vi "Main Loop.vi"(8 "error in (no error)":errorcluster, 10 "Chart Notifier":refnum<notifier>, 11 "Message Queues":T1) -> (0 "error out":errorcluster)   [LabVIEW 2018, in "Scale Module.lvlib" / "Scale Module Engine.lvlib"]
uses:
  Scale Module Engine.lvlib
  Scale Message Queues.ctl
  support/Message Queue/Message Cluster.ctl
  State Cluster.ctl
  State Enum.ctl
  Feed Module/Controls/Scale Module Settings Cluster.ctl
  Mettler Toledo/Controls/Settings Cluster.ctl
  Feed Module/Controls/Scale Module Display.ctl
  <vilib>/Platform/TimedLoop/XDataNode/timing_clust.ctl
  <vilib>/Platform/TimedLoop/XDataNode/nitl_modes.ctl
  <vilib>/Platform/TimedLoop/XDataNode/wakeup.ctl
  Tag VIs/Tag FGV Operation Enum.ctl
  support/Message Queue/Enqueue Message (Single).vi
  <vilib>/Utility/error.llb/Error Cluster From Error Code.vi
  <vilib>/Platform/TimedLoop/XDataNode/XDataNode.xnode
  <vilib>/ErrorRing/Error Ring.xnode
  support/Message Queue/Message Queue.lvlib
  <vilib>/Platform/TimedLoop/XDataNode/XDNodeRunTimeDep.lvlib
  Scale Module.lvlib
  Mettler Toledo/Mettler Toledo.lvlib
  Shared Variables/Dynamic Shared Variables.lvlib
  support/Support Library.lvlib
panel:
  out "Period (s)":dbl format="%_4g"
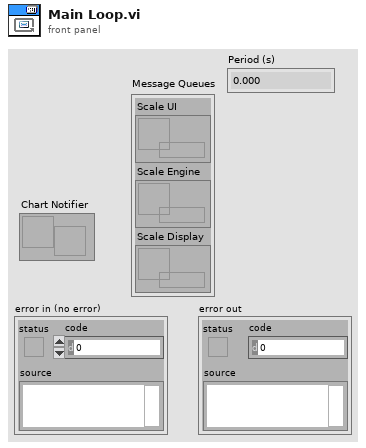
[diagram p1: front panel]
types:
  T1 = typedef "Scale Module.lvlib/Scale Message Queues.ctl" = cluster{"Scale UI":refnum<queue>, "Scale Engine":refnum<queue>, "Scale Display":refnum<queue>}
  T2 = typedef "Scale Module.lvlib/Scale Module Engine.lvlib/State Cluster.ctl" = cluster{"State":T3, "Start Time":timestamp, "Configuration":T4, "Current Time":timestamp, "First Iteration":bool, "Data":cluster{"Scale Read(g)":dbl}, "Process Name":string, "Log Started":bool}
  T3 = typedef "Scale Module.lvlib/Scale Module Engine.lvlib/State Enum.ctl" = enum16{"Measuring", "Idle"}
  T4 = typedef "Scale Module.lvlib/Scale Module Settings Cluster.ctl" = cluster{"Cycle Period":dbl, "Mettler":T5, "Scale Type":string}
  T5 = typedef "Mettler Toledo.lvlib/Settings Cluster.ctl" = cluster{"VISA resource name":refnum<visa-resource-name>, "Simulated?":bool}
  T6 = typedef "XDNodeRunTimeDep.lvlib/timing_clust.ctl" = cluster{"Expected End [f-1]":u64, "Actual End [f-1]":u64, "Finished Late? [f-1]":bool, "Expected End [i-1]":u64, "Actual End [i-1]":u64, "Finished Late? [i-1]":bool, "Expected Start [i]":u64, "Actual Start [i]":u64, "Expected Start [f]":u64, "Actual Start [f]":u64, "Source Name":string, "Structure Name":string, "Period":i64, "Deadline":i64, "Offset":i64, "Start":i64, "Priority":i32, "Timeout":i32, "Mode":T7, "Wakeup Reason":T8, "Error":errorcluster, "Source Type":string, "Secondary Source Type":string, "Global End Time":u64, "Global Start Time":u64, "Frame Duration":u64, "Iteration Duration":u64, "Assigned CPU":i32, "I/O Scan Engine Mode":u32}
  T7 = typedef "XDNodeRunTimeDep.lvlib/nitl_modes.ctl" = enum32{"No Change", "Process missed periods, maintain original phase", "Discard missed periods, maintain original phase", "Process missed periods, ignore original phase", "Discard missed periods, ignore original phase"}
  T8 = typedef "XDNodeRunTimeDep.lvlib/wakeup.ctl" = enum32{"Normal", "Aborted", "Asynchronous wakeup", "Timing source error", "Timed loop error", "Timeout"}
  T9 = cluster{"enable? (F)":bool, "name":string, "alarm on":bool, "priority":u32, "ack type":enum16{"Auto", "User", "None", "Each Occurrence"}, "area":string, "description":string, "log? (T)":bool}
  T10 = typedef "Tag FGV Operation Enum.ctl" = enum16{"Init", "Set Notification Queue", "Create Tag", "Commit", "Write Tag (Numeric)", "Write Tag (Boolean)", "Read All Tags", "Read One Tag", "Delete Tag Category", "Set Alarm Parameters (Numeric)", "Set Alarm Parameters (Boolean)", "Enable All Alarms", "Disable All Alarms", "Delete All Tags", "Read Alarms", "Ack Alarm", "Read Alarm Parameters (Numeric)", "Read Alarm Parameters (Boolean)"}
  T11 = enum32{"u32BitField", "bool", "double", "string", "int8", "uint8", "int16", "uint16", "int32", "uint32", "int64", "uint64", "single", "double waveform", "int16 waveform", "array of boolean", "array of int8", "array of uint8", "array of int16", "array of uint16", "array of int32", "array of uint32", "array of int64", "array of uint64", "array of single", "array of double", "array of double waveform", "array of int16 waveform", "array of string", "variant", "timestamp", "fixed point", "custom"}
  T12 = typedef "Scale Module.lvlib/Scale Module Display.ctl" = cluster{"Scale Value":dbl, "Cycle Period":dbl}
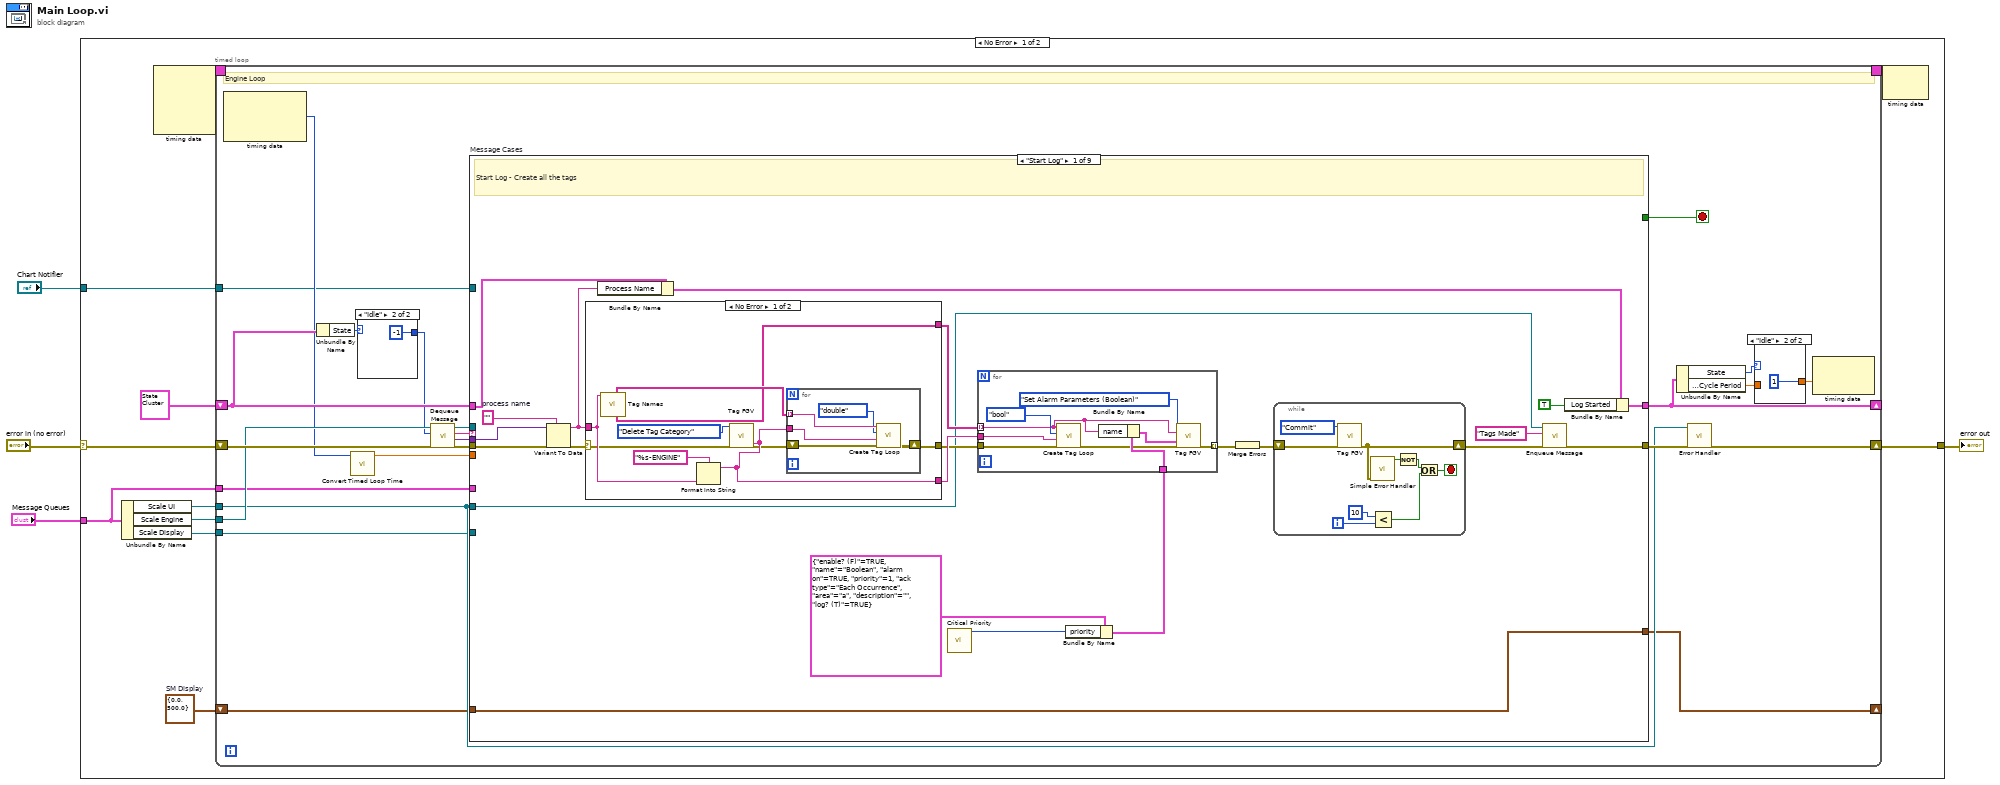
[diagram p0: block diagram]
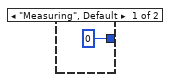
[diagram p3: hidden frame]
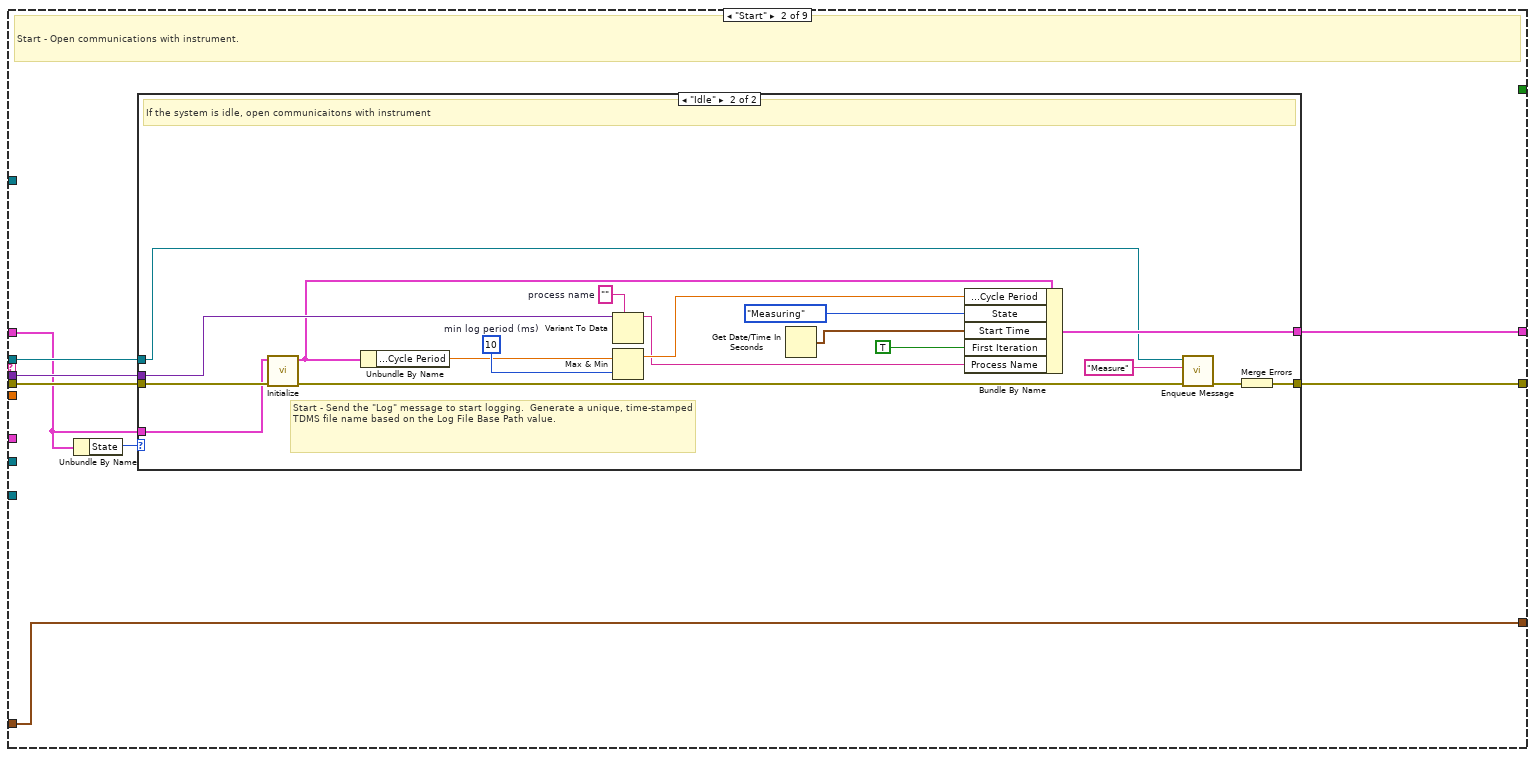
[diagram p5: hidden frame]
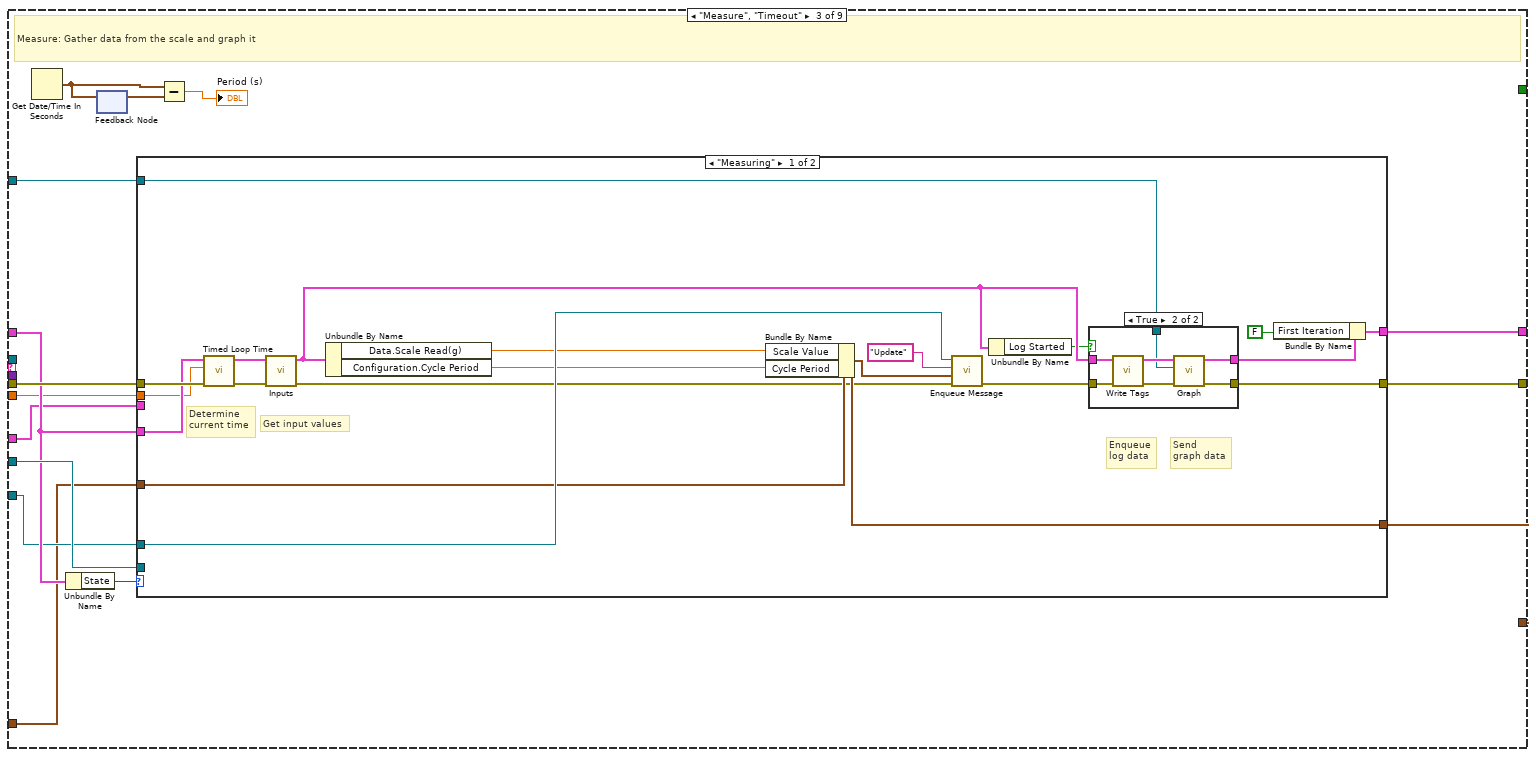
[diagram p7: hidden frame]
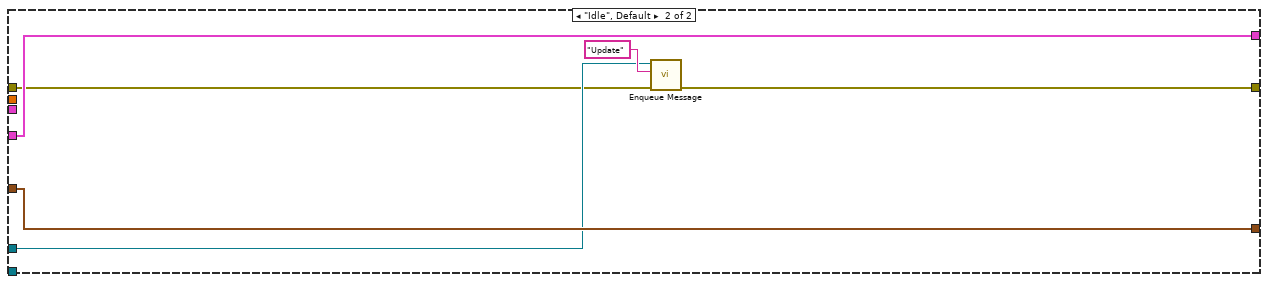
[diagram p9: hidden frame]
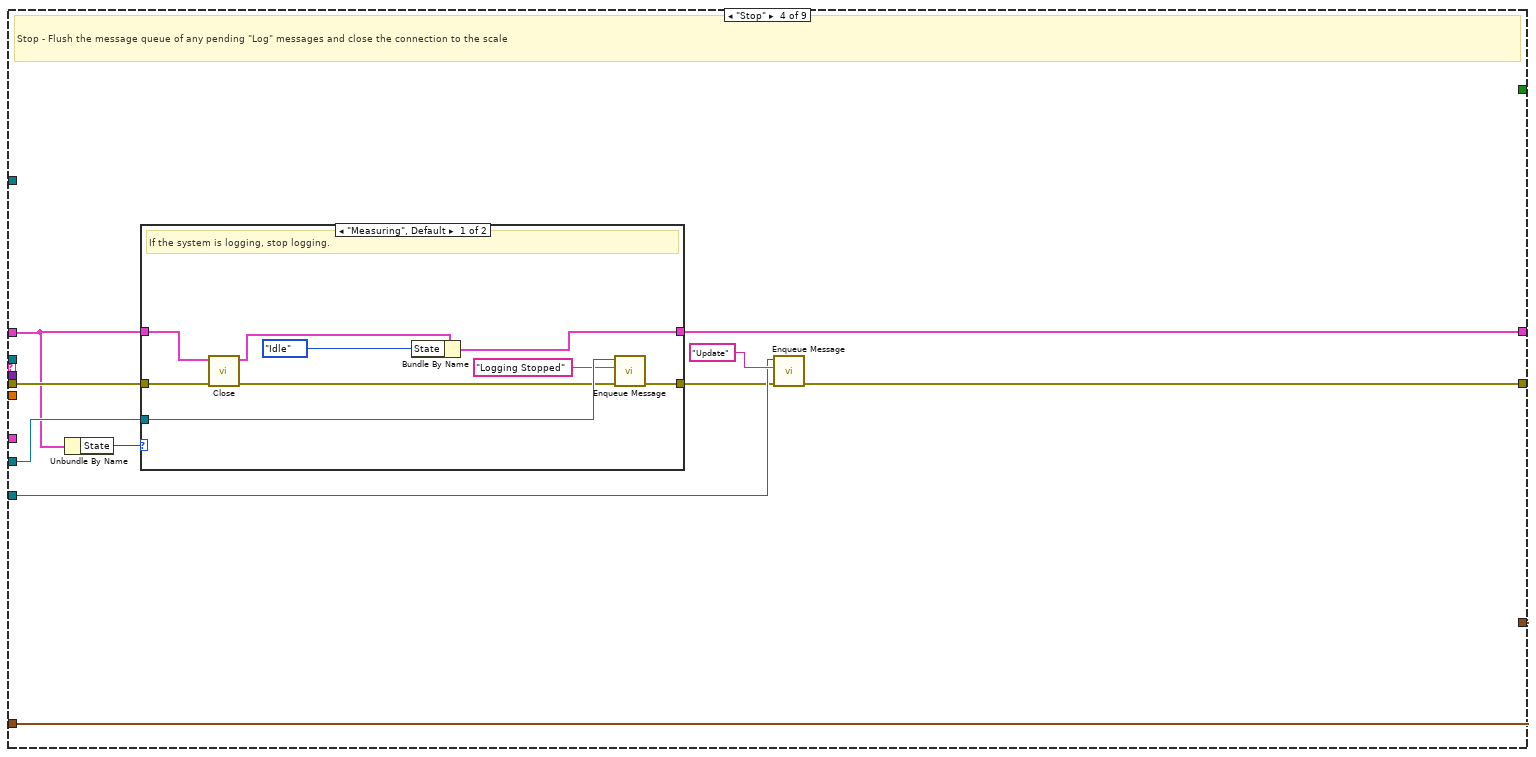
[diagram p10: hidden frame]
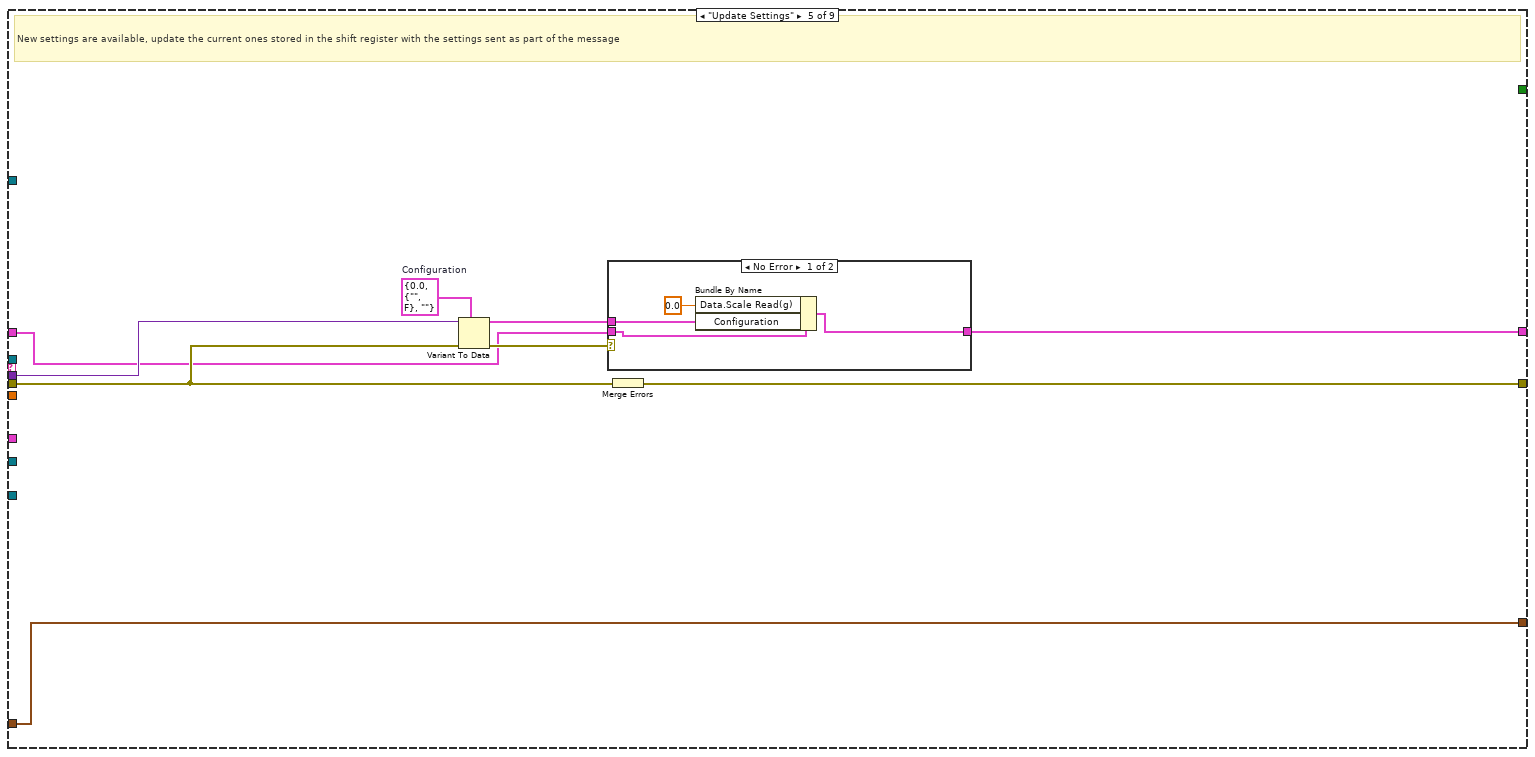
[diagram p12: hidden frame]
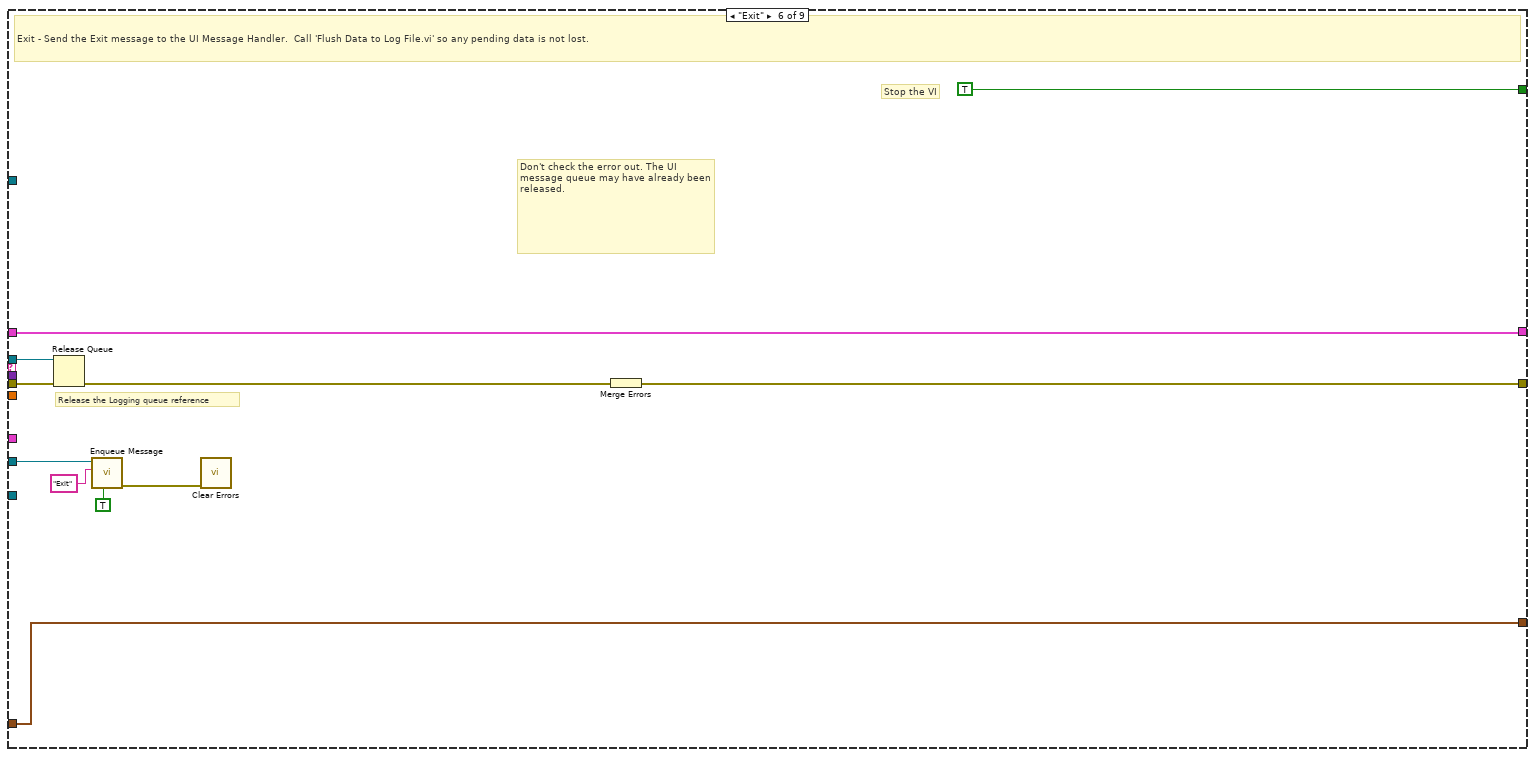
[diagram p14: hidden frame]
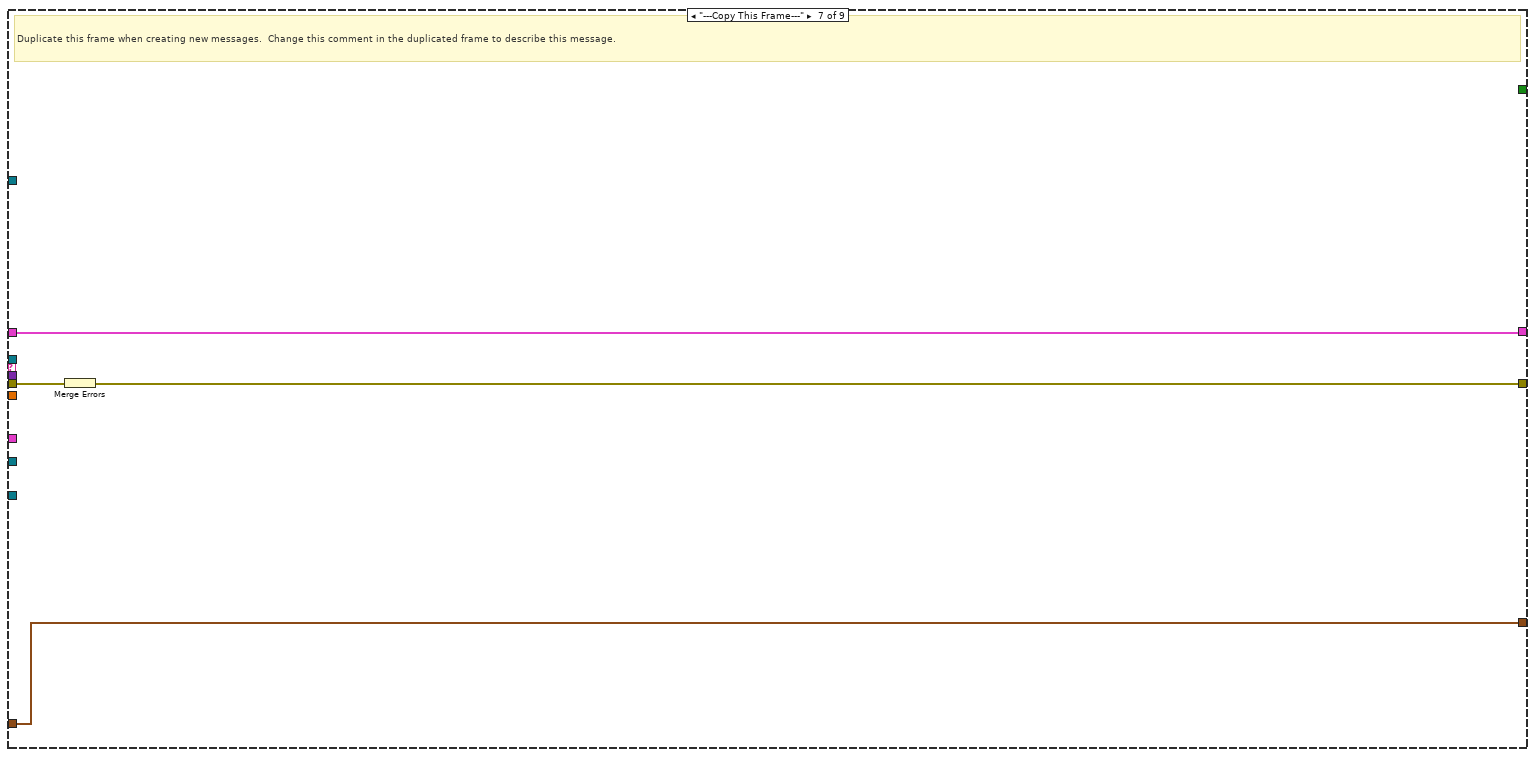
[diagram p15: hidden frame]
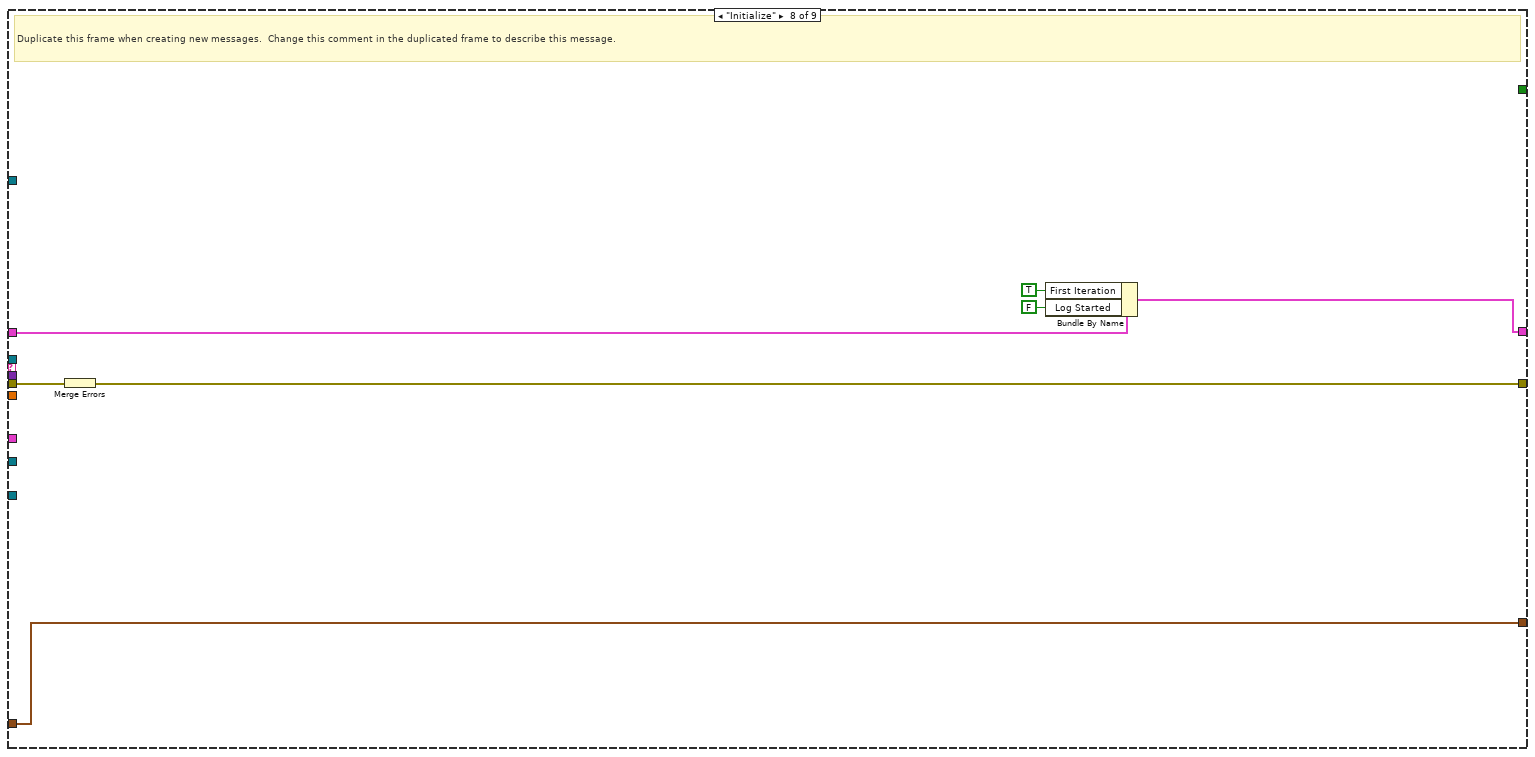
[diagram p16: hidden frame]
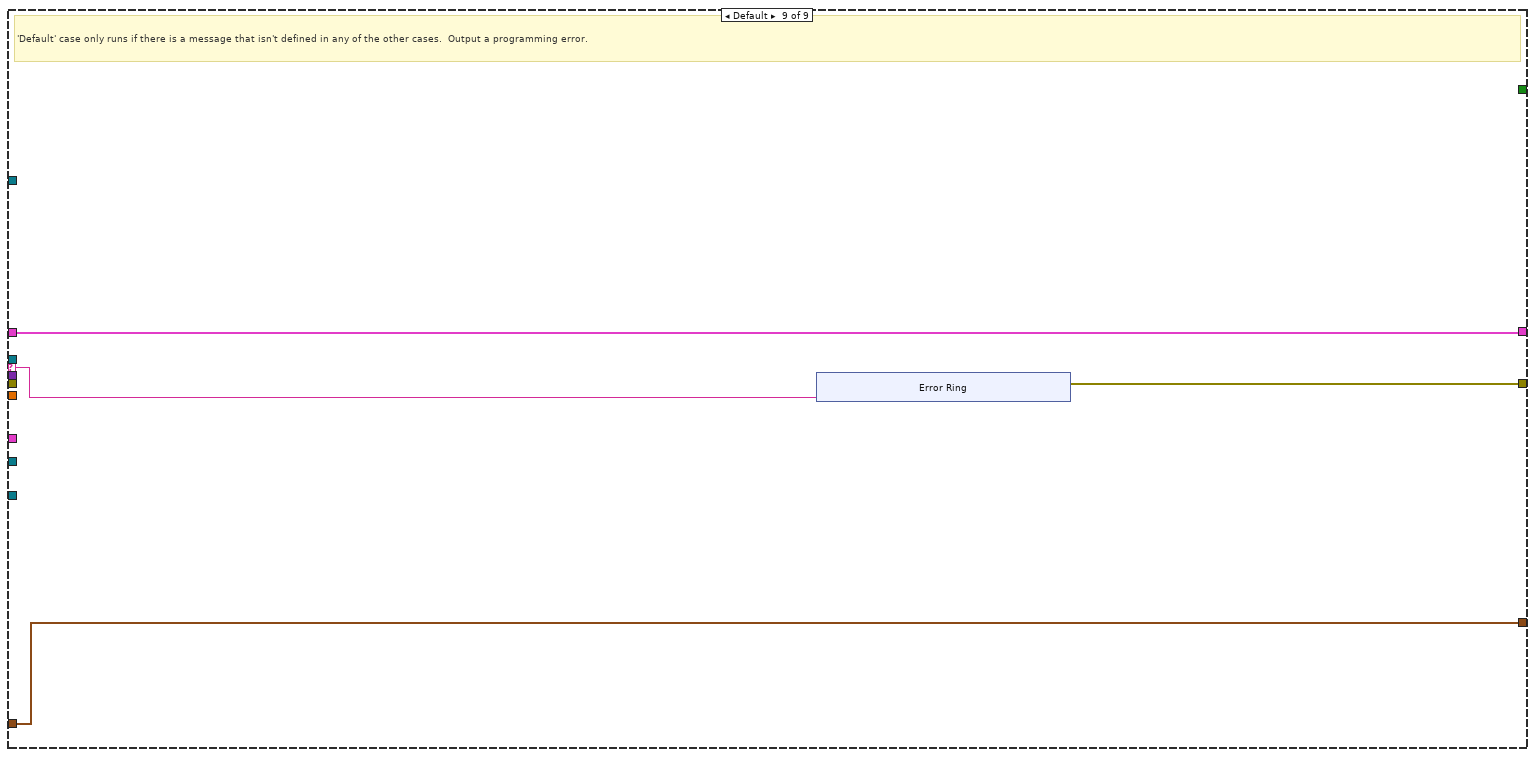
[diagram p17: hidden frame]
diagram:
  n1 = case shown="No Error" "error in (no error)" {
    selector: "error in (no error)" -> [w14 w252]
    tunnel: "Message Queues" -> [w9 _]
    tunnel: [w15 w252] -> w3
    tunnel: "Chart Notifier" -> [w7 _]
    frame No Error {
      w5 = T12 {"Scale Value"=0.0, "Cycle Period"=500.0}  # SM Display
      n2 = Unbundle By Name(w9) -> ("Scale UI"=w13:refnum<queue>, "Scale Engine"=w8:refnum<queue>, "Scale Display"=w6:refnum<queue>)
      n3 = node-c288() -> (w11:T6)  [unwired: 4 in]
      n4 = timed-loop {
        tunnel: w8 -> [w33]
        shift-right: [w17] -> _
        shift-left: T2 {"State"=enum."Idle", "Start Time"=timestamp(0 s since 1904-01-01), "Configuration"={"Cycle Period"=0.0, "Mettler"={"VISA resource name"="", "Simulated?"=FALSE}, "Scale Type"=""}, "Current Time"=timestamp(0 s since 1904-01-01), "First Iteration"=FALSE, "Data"={"Scale Read(g)"=0.0}, "Process Name"="", "Log Started"=FALSE} -> [w29]
        shift-right: [w31] -> w15
        shift-left: w14 -> [w38]
        tunnel: w13 -> [w30]
        timing: w11 -> [_]
        timing-out: [_] -> w10
        tunnel: w9 -> [w21]
        tunnel: w7 -> [w20]
        tunnel: w6 -> [w19]
        shift-right: [w18] -> _
        shift-left: w5 -> [w16]
        stop <- w39 stop-if-true
        # "Engine Loop"
        n5 = node-c288() -> (w23:i64)  [unwired: 1 in, 2 out]
        n6 = Unbundle By Name(w29) -> ("State"=w28:T3)
        n7 = call "Convert Timed Loop Time.vi"("Actual Start [i]"=w23) -> ("ET since start (s)"=w22:dbl)  [unwired: 10 in]
        n8 = case shown="\"Idle\"" w28 {
          tunnel: [0 ("timeout in ms (-1)") -1 ("timeout in ms (-1)")] -> w27
          frame "Measuring", Default {
          }
          frame "Idle" {
          }
        }
        n9 = call "Dequeue Message.vi"("error in (no error)"=w38, "timeout in ms (-1)"=w27, "Message Queue"=w33) -> ("error out"=w37:errorcluster, "Message Data"=w35:variant, "Message"=w36:string, "dup Message Queue"=w34:refnum<queue>)  [unwired: 5 in]
        n10 = case "Message Cases" shown="\"Start Log\"" w36 {
          selector: w36 -> [_ _ _ _ _ _ _ _ w241]
          tunnel: w34 -> [_ w110 _ _ _ w221 _ _ _]
          tunnel: w37 -> [w65 w109 w143 w191 w209 w224 w231 w238 _]
          tunnel: [w52 w111 w144 w182 w211 w226 w230 w237 w242] -> w32
          tunnel: w29 -> [w64 w106 w142 w188 w207 w217 w228 w235 w239]
          tunnel: [_ _ _ _ _ TRUE _ _ _] -> w39
          tunnel: w35 -> [w66 w107 _ _ w210 _ _ _ _]
          tunnel: w30 -> [w51 _ w145 w190 _ w225 _ _ _]
          tunnel: w22 -> [_ _ w141 _ _ _ _ _ _]
          tunnel: w21 -> [_ _ w140 _ _ _ _ _ _]
          tunnel: w20 -> [_ _ w136 _ _ _ _ _ _]
          tunnel: w19 -> [_ _ w135 w184 _ _ _ _ _]
          tunnel: w16 -> [w70 w105 w134 w187 w204 w218 w229 w236 w240]
          tunnel: [w70 w105 w133 w187 w204 w218 w229 w236 w240] -> w18
          tunnel: [w55 w104 w132 w186 w203 w217 w228 w232 w239] -> w17
          frame "Start Log" {
            w69 = ""  # process name
            # "Start Log - Create all the tags"
            n11 = Variant To Data(error in=w65, type=w69, Variant=w66) -> (data=w67:string, error out=w68:errorcluster)
            n12 = case shown="No Error" w68 {
              selector: w68 -> [w91 w103]
              tunnel: [w97 w103] -> w58
              tunnel: w67 -> [w95 _]
              tunnel: [w90 _] -> w60
              tunnel: [w93 _] -> w59
              frame No Error {
                n13 = call "Tag Names.vi"("Process Name"=w95) -> ("All Boolean Tags"=w93:string[], "All  Numeric Tags"=w94:string[])  [unwired: 8 in, 1 out]
                n14 = Format Into String(format string="%s-ENGINE", w95) -> (resulting string=w90:string)  [unwired: 2 in, 1 out]
                n15 = call "Tag FGV.vi"("Operation"=Tag_FGV_Operation_Enum."Delete Tag Category", "error in (no error)"=w91, "Tag Category"=w90) -> ("error out"=w89:errorcluster)  [unwired: 5 in, 7 out]
                n16 = for {
                  shift-right: [w102] -> w97
                  shift-left: w89 -> [w101]
                  tunnel: w90 -> [w98]
                  tunnel: w94 -> [w100] mode=indexing
                  n17 = call "Create Tag Loop.vi"("error in (no error)"=w101, "Tag Category"=w98, "data type"=T11."double", "Tag Name"=w100) -> ("error out"=w102:errorcluster)  [unwired: 7 in]
                }
              }
              frame Error {
              }
            }
            n18 = Bundle By Name(cluster=w64, "Process Name"=w67) -> (w56:T2)
            n19 = call "Critical Priority.vi"() -> ("critical priority"=w62:i32)  [unwired: 11 in]
            n20 = Bundle By Name(cluster=T9 {"enable? (F)"=TRUE, "name"="Boolean", "alarm on"=TRUE, "priority"=1, "ack type"=enum."Each Occurrence", "area"="a", "description"="", "log? (T)"=TRUE} ("Boolean alarm settings"), "priority"=w62) -> (w61:T9)
            n21 = for {
              tunnel: w61 -> [w88]
              tunnel: [w80] -> w57 mode=indexing
              tunnel: w59 -> [w82] mode=indexing
              tunnel: w60 -> [w85]
              tunnel: w58 -> [w87]
              n22 = call "Create Tag Loop.vi"("error in (no error)"=w87, "Tag Category"=w85, "data type"=T11."bool", "Tag Name"=w82) -> ("error out"=w81:errorcluster)  [unwired: 7 in]
              n23 = Bundle By Name(cluster=w88, "name"=w82) -> (w83:T9)
              n24 = call "Tag FGV.vi"("Operation"=Tag_FGV_Operation_Enum."Set Alarm Parameters (Boolean)", "Tag Name"=w82, "Data"=w83, "error in (no error)"=w81) -> ("error out"=w80:errorcluster)  [unwired: 4 in, 7 out]
            }
            n25 = Merge Errors(w57) -> (w49:errorcluster)
            n26 = while {
              shift-right: [w71] -> w50
              shift-left: w49 -> [w72]
              i -> [w78]
              stop <- w74 stop-if-true
              n27 = call "Tag FGV.vi"("Operation"=Tag_FGV_Operation_Enum."Commit", "error in (no error)"=w72) -> ("error out"=w71:errorcluster)  [unwired: 6 in, 7 out]
              n28 = call <vilib>:"Simple Error Handler.vi"("error in (no error)"=w71) -> ("error?"=w79:bool)  [unwired: 4 in, 4 out]
              n29 = Less?(x=10, y=w78) -> (x < y?=w75:bool)
              n30 = Not(x=w79) -> (.not. x?=w76:bool)
              n31 = Or(x=w76, y=w75) -> (x .or. y?=w74:bool)
            }
            n32 = call-poly "Enqueue Message.vi"("error in (no error)"=w50, "Message"="Tags Made", "Message Queue"=w51) -> ("error out"=w52:errorcluster)  [unwired: 7 in, 1 out]
            n33 = Bundle By Name(cluster=w56, "Log Started"=TRUE) -> (w55:T2)
          }
          frame "Start" {
            # "Start - Open communications with instrument."
            n34 = Unbundle By Name(w106) -> ("State"=w108:T3)
            n35 = case shown="\"Idle\"" w108 {
              tunnel: [w112 w131] -> w111
              tunnel: w110 -> [_ w122]
              tunnel: w109 -> [w112 w119]
              tunnel: w106 -> [w113 w118]
              tunnel: [w113 w129] -> w104
              tunnel: w107 -> [_ w116]
              frame "Measuring", Default {
                # "The system is already running. Ignore the \"Start\" message."
              }
              frame "Idle" {
                w117 = ""  # process name
                w126 = 10  # min log period (ms)
                # "Start - Send the \"Log\" message to start logging.  Generate a unique, time-stamped TDMS file name based on the Log File Base Path value."
                # "If the system is idle, open communicaitons with instrument"
                n36 = call "Initialize.vi"("error in (no error)"=w119, "State in"=w118) -> ("error out"=w120:errorcluster, "State out"=w114:T2)  [unwired: 8 in]
                n37 = Unbundle By Name(w114) -> ("Configuration.Cycle Period"=w125:dbl)
                n38 = Variant To Data(type=w117, Variant=w116) -> (data=w115:string)  [unwired: 1 in, 1 out]
                n39 = Max & Min(x=w125, y=w126) -> (max(x,y)=w124:dbl)  [unwired: 1 out]
                n40 = Get Date/Time In Seconds() -> (seconds since 1Jan1904=w123:timestamp)
                n41 = Bundle By Name(cluster=w114, "Configuration.Cycle Period"=w124, "State"=State_Enum."Measuring", "Start Time"=w123, "First Iteration"=TRUE, "Process Name"=w115) -> (w129:T2)
                n42 = call-poly "Enqueue Message.vi"("error in (no error)"=w120, "Message"="Measure", "Message Queue"=w122) -> ("error out"=w127:errorcluster)  [unwired: 7 in, 1 out]
                n43 = Merge Errors(w127) -> (w131:errorcluster)
              }
            }
          }
          frame "Measure", "Timeout" {
            # "Measure: Gather data from the scale and graph it"
            n44 = Get Date/Time In Seconds() -> (seconds since 1Jan1904=w138:timestamp)
            n45 = Unbundle By Name(w142) -> ("State"=w146:T3)
            n46 = feedback-in #1(w138) -> ()
            n47 = feedback #1() -> (w139:timestamp)  [unwired: 1 in]
            n48 = case shown="\"Measuring\"" w146 {
              tunnel: w143 -> [w164 w177]
              tunnel: w142 -> [w162 w180]
              tunnel: w145 -> [_ _]
              tunnel: [w166 w176] -> w144
              tunnel: [w159 w180] -> w132
              tunnel: w141 -> [w161 _]
              tunnel: w140 -> [_ _]
              tunnel: w136 -> [w157 _]
              tunnel: w135 -> [w156 w178]
              tunnel: w134 -> [w154 w181]
              tunnel: [w151 w181] -> w133
              frame "Measuring" {
                # "Determine\ncurrent time"
                # "Send\ngraph data"
                # "Enqueue\nlog data"
                # "Get input values"
                n49 = call "Timed Loop Time.vi"("error in (no error)"=w164, "ET since start (s)"=w161, "State in"=w162) -> ("error out"=w165:errorcluster, "State out"=w163:T2)  [unwired: 7 in]
                n50 = call "Inputs.vi"("error in (no error)"=w165, "State in"=w163) -> ("error out"=w150:errorcluster, "State out"=w148:T2)  [unwired: 8 in]
                n51 = Unbundle By Name(w148) -> ("Data.Scale Read(g)"=w153:dbl, "Configuration.Cycle Period"=w152:dbl)
                n52 = Bundle By Name(cluster=w154, "Scale Value"=w153, "Cycle Period"=w152) -> (w151:T12)
                n53 = call-poly "Enqueue Message.vi"("error in (no error)"=w150, "Message Data"=w151, "Message"="Update", "Message Queue"=w156) -> ("error out"=w149:errorcluster)  [unwired: 6 in, 1 out]
                n54 = Unbundle By Name(w148) -> ("Log Started"=w147:bool)
                n55 = case shown="True" w147 {
                  tunnel: [w167 w173] -> w166
                  tunnel: [w168 w172] -> w160
                  tunnel: w157 -> [_ w171]
                  tunnel: w148 -> [w168 w170]
                  tunnel: w149 -> [w167 w169]
                  frame False {
                  }
                  frame True {
                    n56 = call "Write Tags.vi"("error in (no error)"=w169, "State in"=w170) -> ("error out"=w174:errorcluster, "State out"=w175:T2)  [unwired: 8 in]
                    n57 = call "Graph.vi"("error in (no error)"=w174, "notifier out"=w171, "State in"=w175) -> ("error out"=w173:errorcluster, "State out"=w172:T2)  [unwired: 7 in]
                  }
                }
                n58 = Bundle By Name(cluster=w160, "First Iteration"=FALSE) -> (w159:T2)
              }
              frame "Idle", Default {
                n59 = call-poly "Enqueue Message.vi"("error in (no error)"=w177, "Message"="Update", "Message Queue"=w178) -> ("error out"=w176:errorcluster)  [unwired: 7 in, 1 out]
              }
            }
            n60 = Subtract(x=w138, y=w139) -> (x-y=→"Period (s)":dbl)
          }
          frame "Stop" {
            # "Stop - Flush the message queue of any pending \"Log\" messages and close the connection to the scale"
            n61 = Unbundle By Name(w188) -> ("State"=w189:T3)
            n62 = case shown="\"Measuring\", Default" w189 {
              tunnel: [w196 w202] -> w183
              tunnel: w191 -> [w193 w202]
              tunnel: w190 -> [w200 _]
              tunnel: w188 -> [w194 w201]
              tunnel: [w198 w201] -> w186
              frame "Measuring", Default {
                # "If the system is logging, stop logging."
                n63 = call "Close.vi"("error in (no error)"=w193, "State in"=w194) -> ("error out"=w192:errorcluster, "State out"=w195:T2)  [unwired: 8 in]
                n64 = Bundle By Name(cluster=w195, "State"=State_Enum."Idle") -> (w198:T2)
                n65 = call-poly "Enqueue Message.vi"("error in (no error)"=w192, "Message"="Logging Stopped", "Message Queue"=w200) -> ("error out"=w196:errorcluster)  [unwired: 7 in, 1 out]
              }
              frame "Idle" {
                # "The system is already idle. Ignore the \"Stop\" message."
              }
            }
            n66 = call-poly "Enqueue Message.vi"("error in (no error)"=w183, "Message"="Update", "Message Queue"=w184) -> ("error out"=w182:errorcluster)  [unwired: 7 in, 1 out]
          }
          frame "Update Settings" {
            w205 = T4 {"Cycle Period"=0.0, "Mettler"={"VISA resource name"="", "Simulated?"=FALSE}, "Scale Type"=""}  # Configuration
            # "New settings are available, update the current ones stored in the shift register with the settings sent as part of the message"
            n67 = Variant To Data(error in=w209, type=w205, Variant=w210) -> (data=w206:T4, error out=w208:errorcluster)
            n68 = case shown="No Error" w208 {
              tunnel: w207 -> [w215 w216]
              tunnel: w206 -> [w214 _]
              tunnel: [w213 w216] -> w203
              frame No Error {
                n69 = Bundle By Name(cluster=w215, "Data.Scale Read(g)"=0.0, "Configuration"=w214) -> (w213:T2)
              }
              frame Error {
              }
            }
            n70 = Merge Errors(w209) -> (w211:errorcluster)
          }
          frame "Exit" {
            # "Release the Logging queue reference"
            # "Don't check the error out. The UI message queue may have already been released."
            # "Stop the VI"
            # "Exit - Send the Exit message to the UI Message Handler.  Call 'Flush Data to Log File.vi' so any pending data is not lost."
            n71 = Release Queue(queue=w221, error in (no error)=w224) -> (error out=w220:errorcluster)  [unwired: 1 in, 2 out]
            n72 = call-poly "Enqueue Message.vi"("Priority Message? (F)"=TRUE, "Message"="Exit", "Message Queue"=w225) -> ("error out"=w219:errorcluster)  [unwired: 7 in, 1 out]
            n73 = call <vilib>:"Clear Errors.vi"("error in (no error)"=w219) -> ()  [unwired: 5 in, 2 out]
            n74 = Merge Errors(w220) -> (w226:errorcluster)
          }
          frame "---Copy This Frame---" {
            # "Duplicate this frame when creating new messages.  Change this comment in the duplicated frame to describe this message."
            n75 = Merge Errors(w231) -> (w230:errorcluster)
          }
          frame "Initialize" {
            # "Duplicate this frame when creating new messages.  Change this comment in the duplicated frame to describe this message."
            n76 = Merge Errors(w238) -> (w237:errorcluster)
            n77 = Bundle By Name(cluster=w235, "First Iteration"=TRUE, "Log Started"=FALSE) -> (w232:T2)
          }
          frame Default {
            # "'Default' case only runs if there is a message that isn't defined in any of the other cases.  Output a programming error."
            n78 = xnode "Error Ring"("parameter 0"=w241) -> ("error out"=w242:errorcluster)
          }
        }
        n79 = Unbundle By Name(w17) -> ("State"=w26:T3, "Configuration.Cycle Period"=w24:dbl)
        n80 = call "Error Handler.vi"("error in (no error)"=w32, "Message Queue"=w30) -> ("dup error in"=w31:errorcluster)  [unwired: 8 in, 1 out]
        n81 = case shown="\"Idle\"" w26 {
          tunnel: [w40 1] -> w25
          tunnel: w24 -> [w40 _]
          frame "Measuring" {
          }
          frame "Idle" {
          }
        }
        n82 = node-c288(w25) -> ()  [unwired: 1 in, 1 out]
      }
      n83 = node-c288(w10) -> ()  [unwired: 1 out]
    }
    frame Error {
    }
  }
  "error out" <- w3
